vi "PID sichtbar machen.vi"(8 "error in (no error)":errorcluster caption="Fehler (Eingang, kein Fehler)", 11 "PID-Parameter Anzeige":refnum<vi>) -> (0 "error out":errorcluster caption="Fehler (Ausgang)")   [LabVIEW 2020, in "Erweiterte Konfig.lvlib"]
uses:
  Erweiterte Konfig.lvlib
  PID-Parameter Anzeige.ctl
  PID-Parameter.ctl
  Visualisierungs Elemente/Zahlen-Eingabefeld.ctl
  <vilib>/Utility/miscctls.llb/LVPositionTypeDef.ctl
panel:
  # "sec"
  # "sec"
  # "°C"
  # "%"
  # "sec"
  # "sec"
  # "°C"
  # "%"
  # "sec"
  # "sec"
  # "°C"
  # "%"
  # "sec"
  # "sec"
  # "°C"
  # "%"
  # "sec"
  # "sec"
  # "°C"
  # "%"
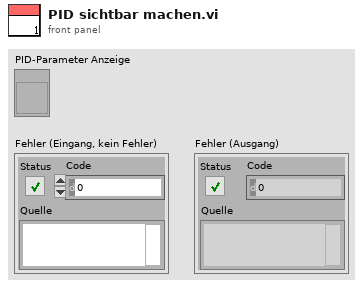
[diagram p1: front panel]
types:
  T1 = typedef "LVPositionTypeDef.ctl" = cluster{"Left":i32, "Top":i32}
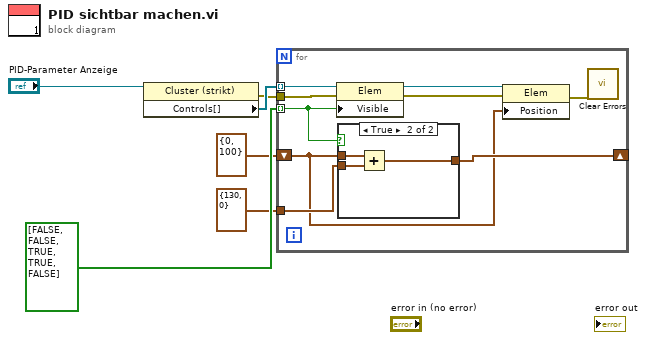
[diagram p0: block diagram]
diagram:
  n1 = property class="Cluster (strikt)"(reference="PID-Parameter Anzeige") -> (error out=w2:errorcluster, "Controls[]"=w3:refnum<vi>[])  [unwired: 1 in, 1 out]
  n2 = for {
    tunnel: bool[] [FALSE, FALSE, TRUE, TRUE, FALSE] -> [w12] mode=indexing
    tunnel: T1 {"Left"=130, "Top"=0} ("Position") -> [w13]
    tunnel: w3 -> [w11] mode=indexing
    shift-right: [w10] -> _
    shift-left: T1 {"Left"=0, "Top"=100} ("Position") -> [w9]
    tunnel: w2 -> [w7]
    n3 = property class="Elem"(reference=w11, error in=w7, "Visible"=w12) -> (reference out=w15:refnum<vi>, error out=w14:errorcluster)
    n4 = case shown="True" w12 {
      tunnel: w13 -> [_ w19]
      tunnel: w9 -> [w16 w18]
      tunnel: [w16 w17] -> w10
      frame False {
      }
      frame True {
        n5 = Add(x=w18, y=w19) -> (x+y=w17:T1)
      }
    }
    n6 = property class="Elem"(reference=w15, error in=w14, "Position"=w9) -> (error out=w8:errorcluster)  [unwired: 1 out]
    n7 = call <vilib>:"Clear Errors.vi"("error in (no error)"=w8) -> ()  [unwired: 5 in, 2 out]
  }
